vi "Excel Get Data.vi"   [LabVIEW 2017, in "NI_ReportGenerationToolkit.lvlib"]
doc: "Retrieves data from the current worksheet. The data type you wire to the <B>data type</B> input determines the polymorphic instance to use."
uses:
  <vilib>/addons/_office/NI_ReportGenerationToolkit.lvlib
  <vilib>/Utility/NIReport.llb/Excel/NI_Excel.lvclass
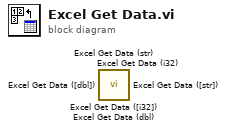
[diagram p0: block diagram]
diagram:
  n1 = call <vilib>:"Excel Get Data ([i32]).vi"() -> ()  [unwired: 13 in, 3 out]
  n2 = call <vilib>:"Excel Get Data (i32).vi"() -> ()  [unwired: 13 in, 3 out]
  n3 = call <vilib>:"Excel Get Data ([dbl]).vi"() -> ()  [unwired: 13 in, 3 out]
  n4 = call <vilib>:"Excel Get Data ([str]).vi"() -> ()  [unwired: 13 in, 3 out]
  n5 = call <vilib>:"Excel Get Data (dbl).vi"() -> ()  [unwired: 13 in, 3 out]
  n6 = call <vilib>:"Excel Get Data (str).vi"() -> ()  [unwired: 13 in, 3 out]
